vi "Calcolo sbilanciamento.vi"(9 "Numeric 1":dbl, 10 "Numeric 2":dbl, 11 "Numeric 3":dbl) -> (3 "sbil%":dbl)   [LabVIEW 2019]
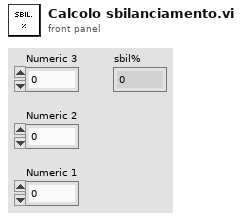
[diagram p1: front panel]
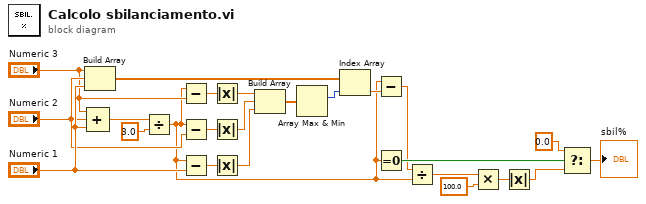
[diagram p0: block diagram]
diagram:
  n1 = Build Array("Numeric 3", "Numeric 2", "Numeric 1") -> (w11:dbl[])
  n2 = Compound Arithmetic op=ADD("Numeric 3", "Numeric 2", "Numeric 1") -> (w2:dbl)
  n3 = Divide(x=w2, y=3.0) -> (x/y=w1:dbl)
  n4 = Subtract(x=w1, y="Numeric 3") -> (x-y=w4:dbl)
  n5 = Subtract(x=w1, y="Numeric 2") -> (x-y=w5:dbl)
  n6 = Subtract(x=w1, y="Numeric 1") -> (x-y=w6:dbl)
  n7 = Absolute Value(x=w4) -> (abs(x)=w7:dbl)
  n8 = Absolute Value(x=w5) -> (abs(x)=w8:dbl)
  n9 = Absolute Value(x=w6) -> (abs(x)=w9:dbl)
  n10 = Build Array(w7, w8, w9) -> (w10:dbl[])
  n11 = Array Max & Min(array=w10) -> (max index (indices)=w12:i32)  [unwired: 3 out]
  n12 = Index Array(array=w11, index=w12) -> (element=w13:dbl)
  n13 = Subtract(x=w1, y=w13) -> (x-y=w14:dbl)
  n14 = Equal To 0?(x=w1) -> (x = 0?=w21:bool)
  n15 = Divide(x=w14, y=w1) -> (x/y=w17:dbl)
  n16 = Multiply(x=w17, y=100.0) -> (x*y=w16:dbl)
  n17 = Absolute Value(x=w16) -> (abs(x)=w23:dbl)
  n18 = Select(t=0.0, s=w21, f=w23) -> (s? t:f=→"sbil%":dbl)
